vi "replaceNameToken.vi"(8 "error in (no error)":errorcluster, 10 "Query In":string, 11 "Goal in":refnum<class "Goal.lvclass">) -> (0 "error out":errorcluster, 2 "Query Out":string, 3 "Goal out":refnum<class "Goal.lvclass">)   [LabVIEW 2018, in "Goal.lvclass"]
uses:
  Goal.lvclass
  Goal.lvclass/Goal.ctl
  Category/Category.lvclass
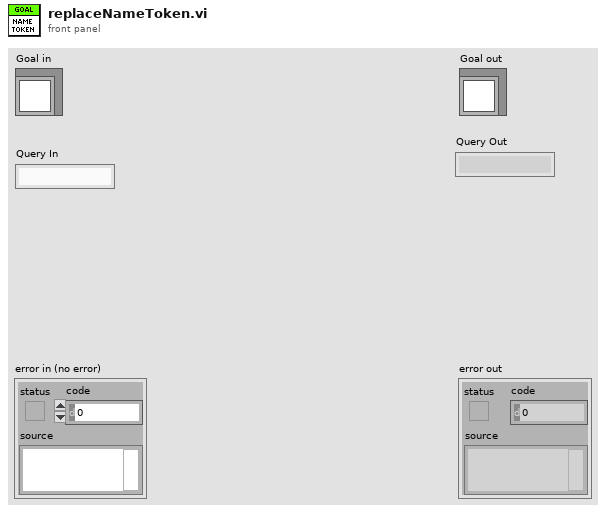
[diagram p1: front panel]
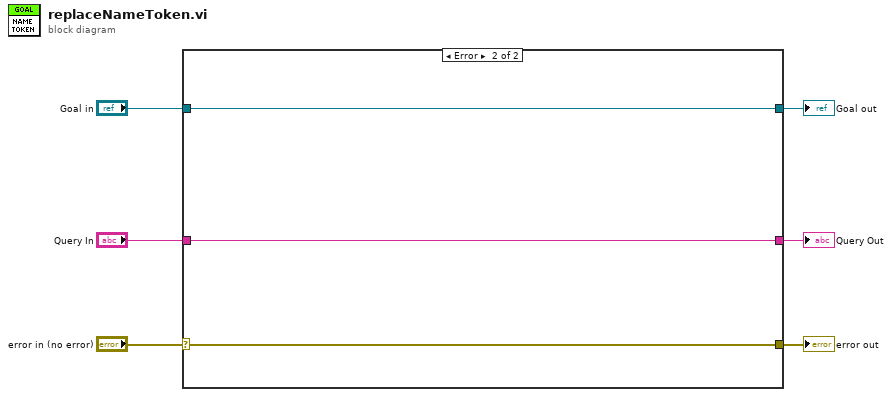
[diagram p0: block diagram]
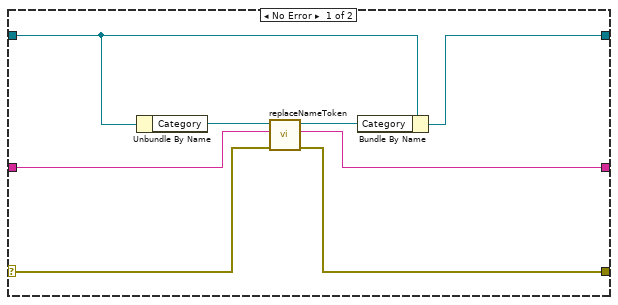
[diagram p2: hidden frame]
diagram:
  n1 = case shown="Error" "error in (no error)" {
    selector: "error in (no error)" -> [w10 w17]
    tunnel: [w9 w17] -> w5
    tunnel: [w13 w16] -> w3
    tunnel: "Goal in" -> [w14 w16]
    tunnel: "Query In" -> [w8 w15]
    tunnel: [w7 w15] -> w1
    frame No Error {
      n2 = Unbundle By Name(w14) -> ("Category"=w12:refnum<class "Category.lvclass">)
      n3 = call "replaceNameToken.vi"("error in (no error)"=w10, "Query In"=w8, "Category in"=w12) -> ("error out"=w9:errorcluster, "Query Out"=w7:string, "Category out"=w11:refnum<class "Category.lvclass">)  [unwired: 6 in]
      n4 = Bundle By Name(cluster=w14, "Category"=w11) -> (w13:refnum<class "Goal.lvclass">)
    }
    frame Error {
    }
  }
  "error out" <- w5
  "Goal out" <- w3
  "Query Out" <- w1
